vi "Set OP and Post OP Measurements.vi"(8 "error in (no error)":errorcluster, 11 "ModSweep in":refnum<class "ModSweep.lvclass">) -> (0 "error out":errorcluster, 3 "ModSweep out":refnum<class "ModSweep.lvclass">)   [LabVIEW 2018, in "ModSweep.lvlib" / "ModSweep.lvclass"]
uses:
  ModSweep.lvclass
  Plugins/Measurements/Servo MSMT.lvlibp/Servo MSMT.lvclass
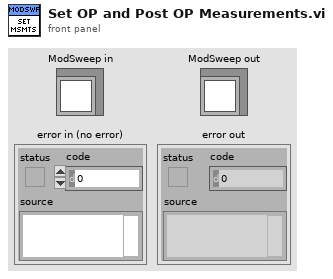
[diagram p1: front panel]
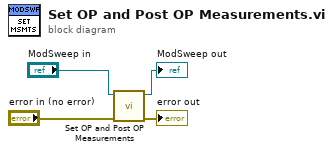
[diagram p0: block diagram]
diagram:
  n1 = call-parent "Set OP and Post OP Measurements.vi"("error in (no error)"="error in (no error)", "Servo MSMT in"="ModSweep in") -> ("error out"=→"error out":errorcluster, "Servo MSMT out"=→"ModSweep out":refnum<class "ModSweep.lvclass">)  [unwired: 8 in]
